vi "_CSMQFGV.vi"(6 "Operation":T3, 8 "Error in":errorcluster caption="Error in (no error)", 9 "create if not found? (T)":bool=TRUE, 11 "Name(\"\" to use uuid) in":string) -> (0 "Error out":errorcluster, 1 "Boolean":bool, 2 "Name":string[](array[string]), 3 "Array":T1[](array[typedef]))   [LabVIEW 2014, in "Communicable State Machine.lvlib"]
uses:
  Communicable State Machine.lvlib
  _CSMQFGVOPER.ctl
  _CSMObj.ctl
  Priority Queue/Priority Queue.lvclass
  Typedef/_CSM_MODE.ctl
  Typedef/_CSM Status Change Event Data.ctl
  Priority Queue/Priority Queue.lvclass/Priority Queue.ctl
  FGV-BroadcastRegistry/Operation-BroadcastRegistry.ctl
  FGV-BroadcastRegistry/global-CSMQ FGV Change Flag.vi
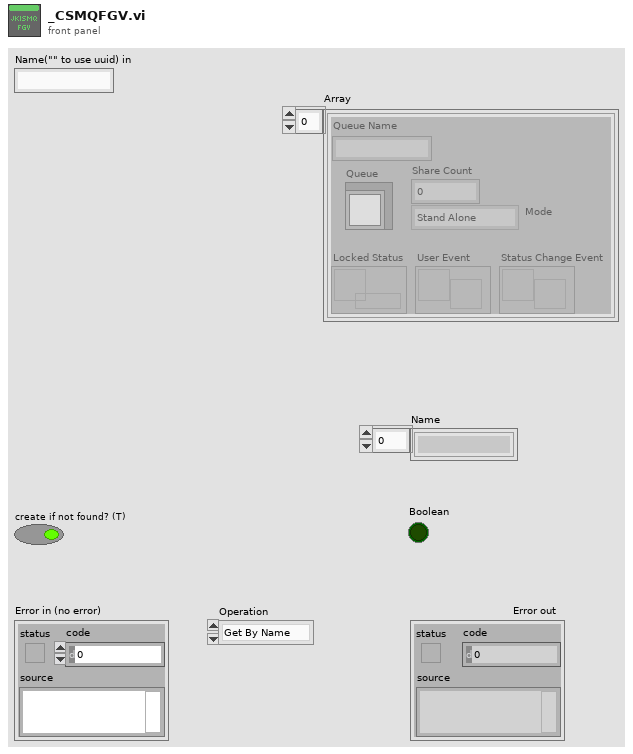
[diagram p1: front panel]
types:
  T1 = typedef "Communicable State Machine.lvlib/_CSMObj.ctl" = cluster{"Queue Name":string, "Mode":T2, "Share Count":i32, "Queue":refnum<class "Priority Queue.lvclass">, "Locked Status":refnum<data-value>, "User Event":refnum<user-event>, "Status Change Event":refnum<user-event>}
  T2 = typedef "Communicable State Machine.lvlib/_CSM_MODE.ctl" = enum16{"Stand Alone", "CSM", "Action Worker"}
  T3 = typedef "Communicable State Machine.lvlib/_CSMQFGVOPER.ctl" = enum16{"Get By Name", "List", "Check If Name Exists", "Release", "Module Status", "Create Status Event Handler", "Destroy Status Event Handler"}
  T4 = typedef "Communicable State Machine.lvlib/Operation-BroadcastRegistry.ctl" = enum16{"Delete Source Module", "Delete Target Module", "Remove Module", "Register", "Unregister", "Check"}
  T5 = typedef "Communicable State Machine.lvlib/_CSM Status Change Event Data.ctl" = cluster{"ModuleName":string, "Status":string, "Arguments":string}
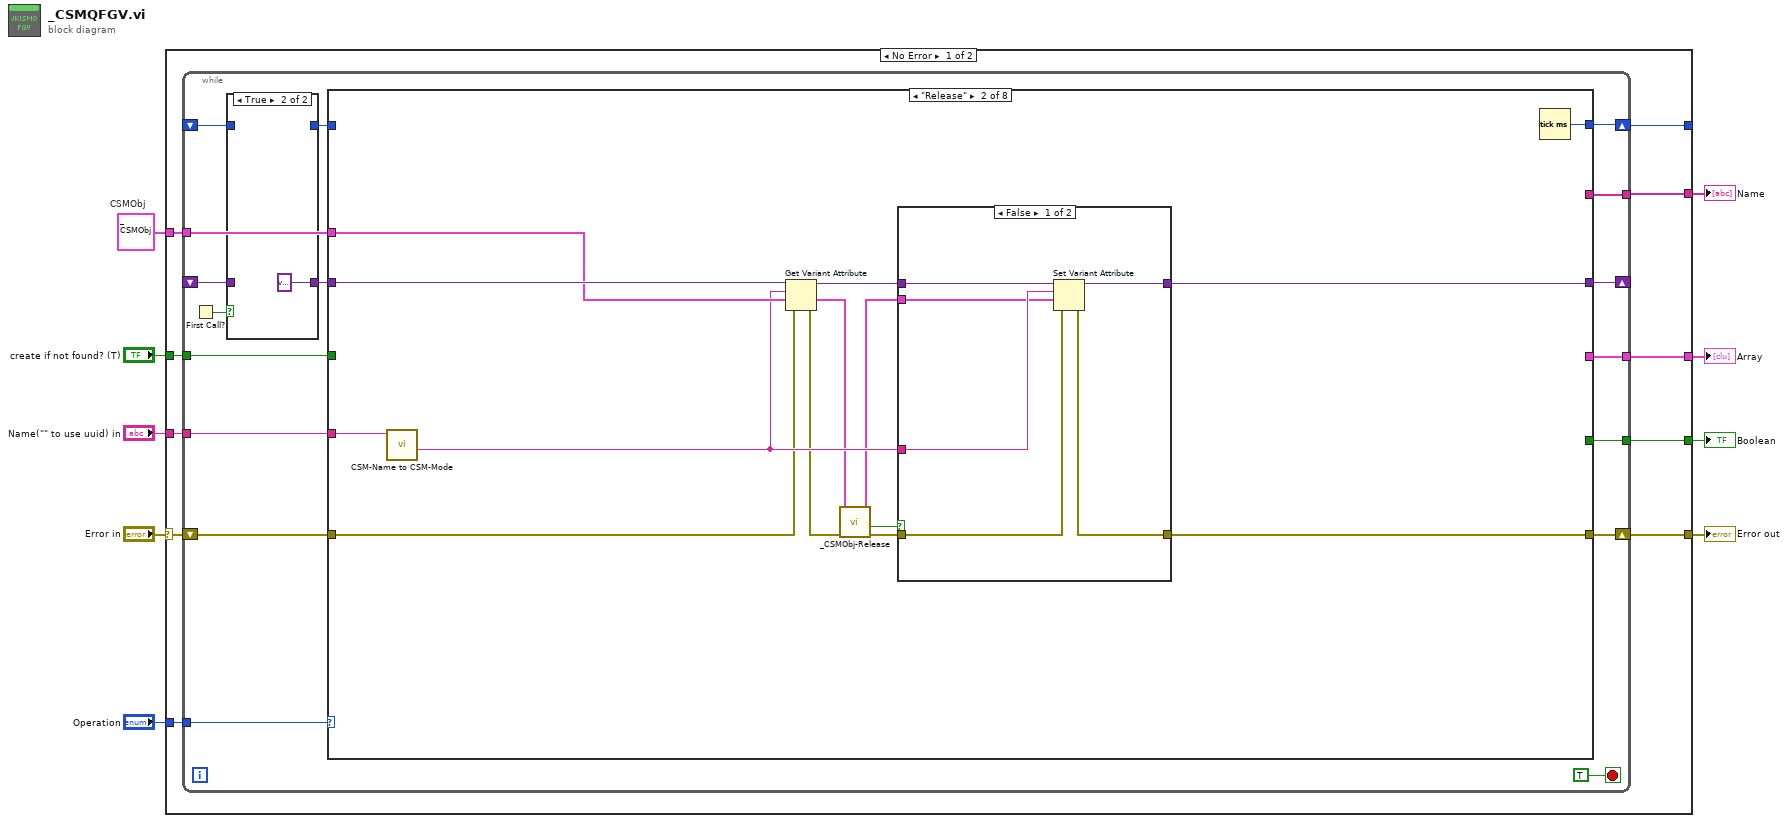
[diagram p0: block diagram]
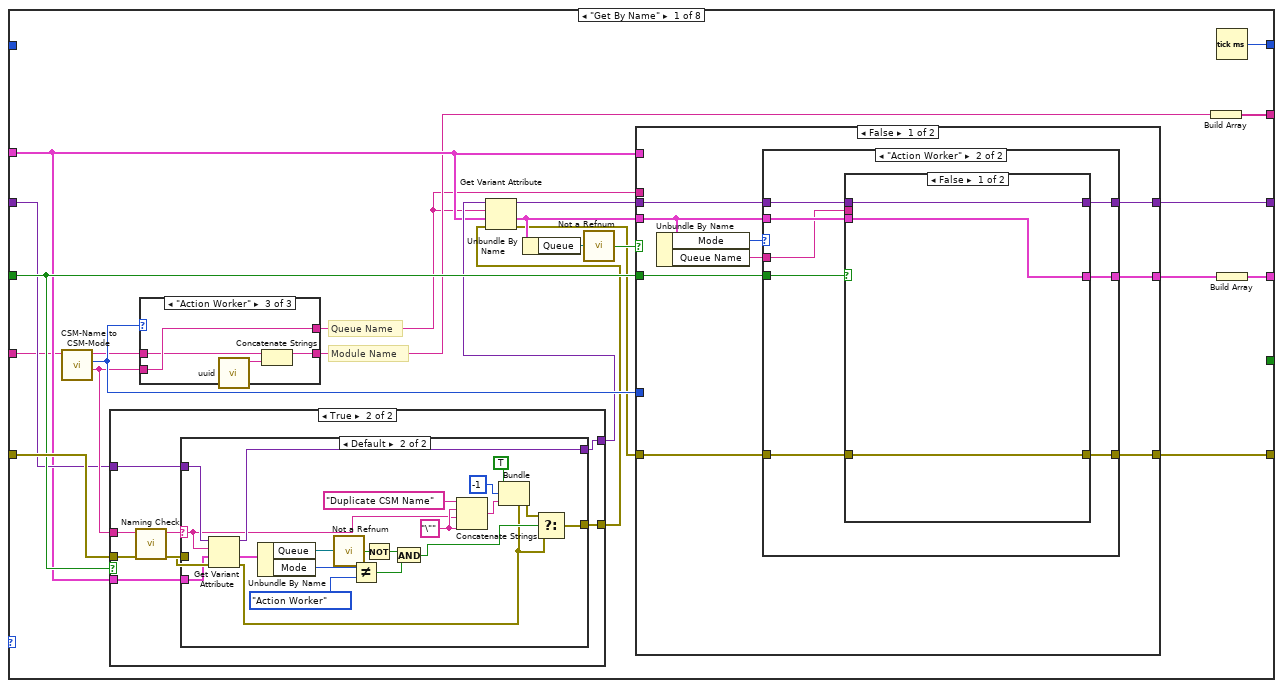
[diagram p3: hidden frame]
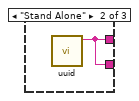
[diagram p7: hidden frame]
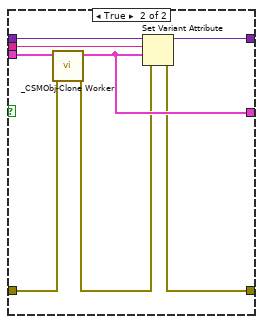
[diagram p9: hidden frame]
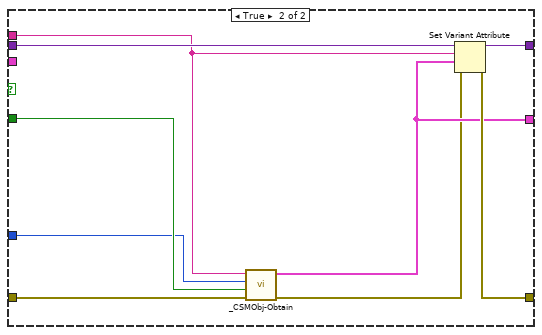
[diagram p10: hidden frame]
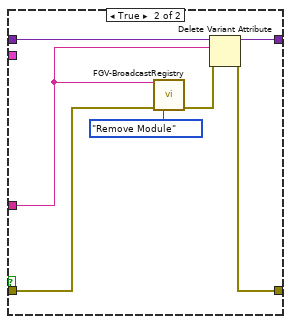
[diagram p11: hidden frame]
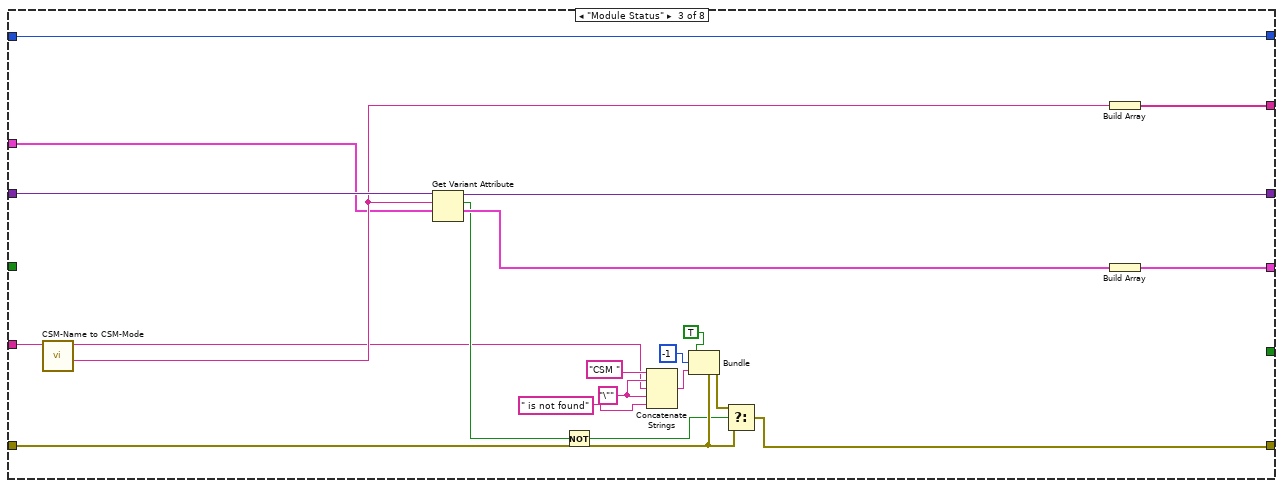
[diagram p12: hidden frame]
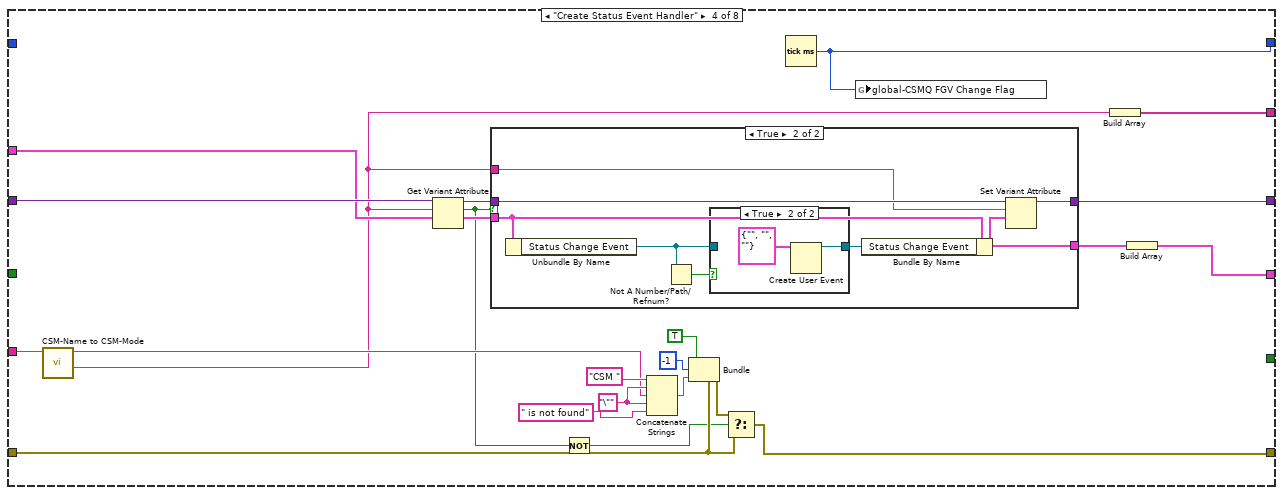
[diagram p13: hidden frame]
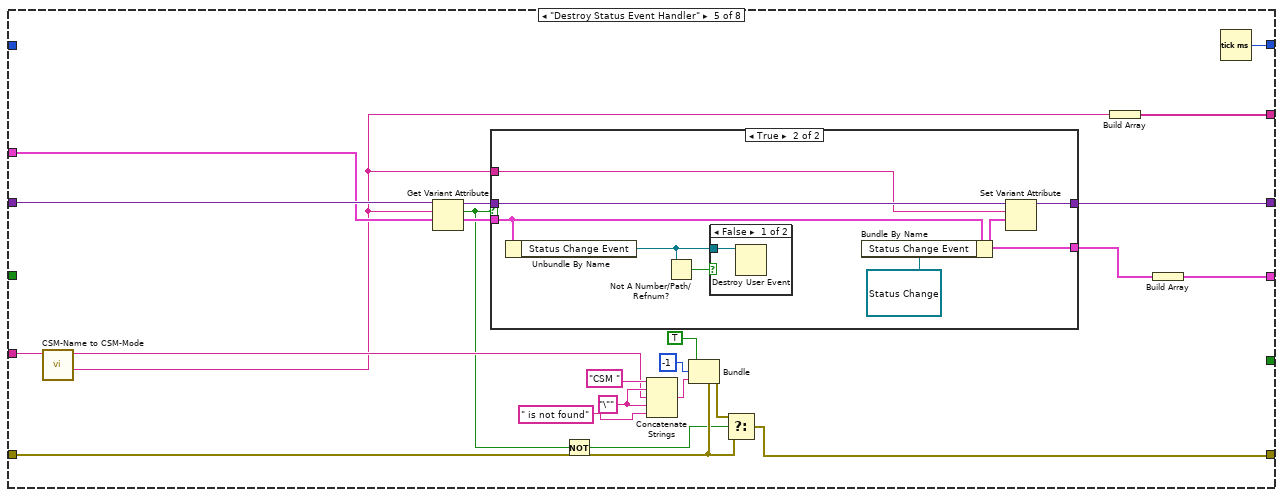
[diagram p16: hidden frame]
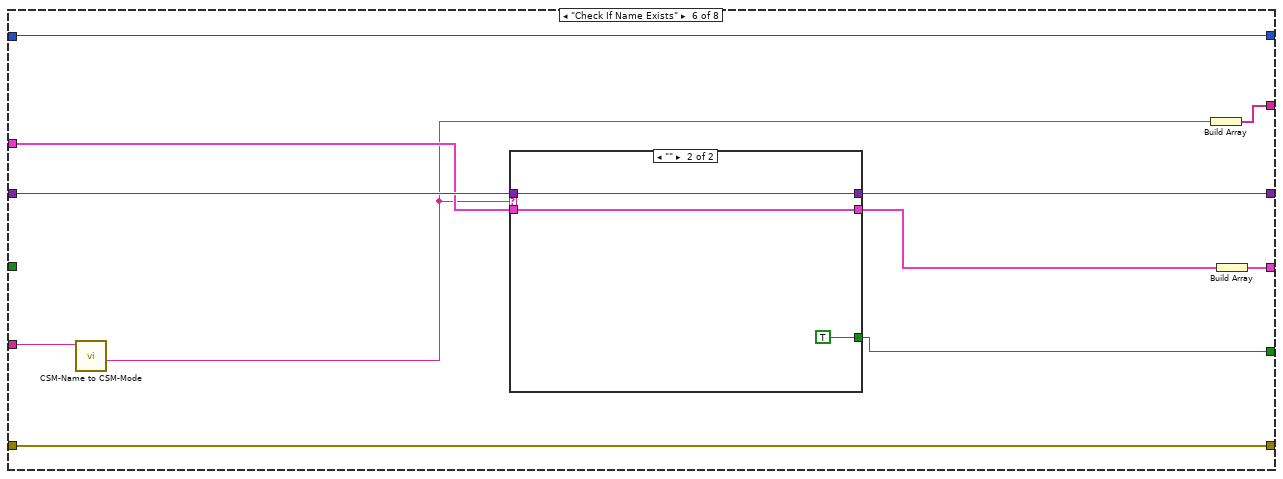
[diagram p19: hidden frame]
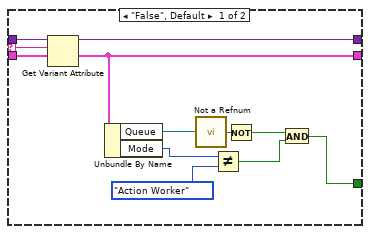
[diagram p20: hidden frame]
diagram:
  w3 = T1 {"Queue Name"="", "Mode"=enum."Stand Alone", "Share Count"=0, "Queue"=refnum, "Locked Status"=refnum, "User Event"=refnum, "Status Change Event"=refnum}  # CSMObj
  n1 = case shown="No Error" "Error in" {
    selector: "Error in" -> [w16 w340]
    tunnel: "Operation" -> [w19 _]
    tunnel: "Name(\"\" to use uuid) in" -> [w18 _]
    tunnel: "create if not found? (T)" -> [w17 _]
    tunnel: [w15 w340] -> w5
    tunnel: [w14 _] -> w4
    tunnel: w3 -> [w13 _]
    tunnel: [w12 _] -> w2
    tunnel: [w11 _] -> w1
    tunnel: [w10 _] -> _
    frame No Error {
      n2 = while {
        tunnel: w19 -> [w35]
        tunnel: w18 -> [w34]
        tunnel: w17 -> [w33]
        tunnel: [w32] -> w12
        shift-right: [w28] -> _
        shift-left: _ -> [w30]
        shift-right: [w26] -> w15
        shift-left: w16 -> [w27]
        tunnel: [w25] -> w14
        tunnel: w13 -> [w24]
        tunnel: [w23] -> w11
        shift-right: [w22] -> w10
        shift-left: _ -> [w20]
        stop <- TRUE stop-if-true
        n3 = First Call?() -> (First Call?: T/F=w31:bool)
        n4 = case shown="True" w31 {
          tunnel: [w38 variant] -> w29
          tunnel: w30 -> [w38 _]
          tunnel: [w37 _] -> w21
          tunnel: w20 -> [w37 _]
          frame False {
          }
          frame True {
          }
        }
        n5 = case shown="\"Release\"" w35 {
          tunnel: w34 -> [w42 w152 w188 w211 w247 w262 _ _]
          tunnel: w33 -> [w48 _ _ _ _ _ w293 _]
          tunnel: [w55 _ w185 w191 w227 w265 w288 _] -> w32
          tunnel: w29 -> [w47 w155 w189 w212 w248 w270 w301 w339]
          tunnel: [w60 w154 w187 w194 w230 w269 w300 w339] -> w28
          tunnel: w27 -> [w50 w149 w176 w203 w239 w267 w298 w338]
          tunnel: [w56 w148 w173 w201 w237 w267 w297 w338] -> w26
          tunnel: [w54 _ w183 w209 w245 w264 w289 _] -> w25
          tunnel: w24 -> [w45 w153 w181 w208 w244 w266 w299 _]
          tunnel: [_ _ _ _ _ w263 _ _] -> w23
          tunnel: w21 -> [_ _ w182 _ _ w260 w295 w337]
          tunnel: [w51 w150 w182 w190 w226 w260 w295 w337] -> w22
          frame "Get By Name" {
            # "Module Name"
            # "Queue Name"
            n6 = call "CSM-Name to CSM-Mode.vi"("String"=w42) -> ("Queue Name"=w49:string, "CSM Mode"=w53:T2, "String(dup)"=w52:string)  [unwired: 8 in]
            n7 = case shown="True" w48 {
              tunnel: w49 -> [_ w66]
              tunnel: [w64 w72] -> w44
              tunnel: w50 -> [w64 w68]
              tunnel: w47 -> [w63 w71]
              tunnel: [w63 w70] -> w46
              tunnel: w45 -> [_ w69]
              frame False {
              }
              frame True {
                n8 = call "Naming Check.vi"("error in (no error)"=w68, "Name(\"\" to use uuid)"=w66) -> ("error out"=w67:errorcluster, "Name(dup)"=w65:string)  [unwired: 8 in]
                n9 = case shown="Default" w65 {
                  selector: w65 -> [_ w75]
                  tunnel: [w73 w95] -> w72
                  tunnel: w67 -> [w73 w78]
                  tunnel: w71 -> [w74 w80]
                  tunnel: [w74 w79] -> w70
                  tunnel: w69 -> [_ w76]
                  frame "", "PostMessageAPI", "SendMessageAPI" {
                  }
                  frame Default {
                    w89 = "\"" ("string")
                    n10 = Get Variant Attribute(Variant=w80, name=w75, default value (empty Variant)=w76, error in=w78) -> (duplicate Variant=w79:variant, value=w82:T1, error out=w77:errorcluster)  [unwired: 1 out]
                    n11 = Unbundle By Name(w82) -> ("Queue"=w83:refnum<class "Priority Queue.lvclass">, "Mode"=w86:T2)
                    n12 = call "Not a Refnum.vi"("Priority Queue.lvclass"=w83) -> ("NaN/Path/Refnum?"=w84:bool)  [unwired: 4 in]
                    n13 = Not Equal?(x=w86, y=_CSM_MODE."Action Worker") -> (x != y?=w88:bool)
                    n14 = Not(x=w84) -> (.not. x?=w85:bool)
                    n15 = And(x=w85, y=w88) -> (x .and. y?=w81:bool)
                    n16 = Concatenate Strings("Duplicate CSM Name" ("String to Prepend to source (\"\")"), w89, w75, w89) -> (w90:string)
                    n17 = Bundle(cluster=w77, "status"=TRUE, "code"=-1, "source"=w90) -> (w94:errorcluster)
                    n18 = Select(t=w94, s=w81, f=w77) -> (s? t:f=w95:errorcluster)
                  }
                }
              }
            }
            n19 = case shown="\"Action Worker\"" w53 {
              tunnel: [w96 w97 w101] -> w40
              tunnel: [w96 w97 w98] -> w41
              tunnel: w52 -> [w96 _ w100]
              tunnel: w49 -> [_ _ w101]
              frame "CSM" {
              }
              frame "Stand Alone" {
                n20 = call "uuid.vi"() -> ("UUID"=w97:string)  [unwired: 11 in]
              }
              frame "Action Worker" {
                n21 = call "uuid.vi"() -> ("UUID"=w99:string)  [unwired: 11 in]
                n22 = Concatenate Strings(w100, w99) -> (w98:string)
              }
            }
            n23 = Get Variant Attribute(Variant=w46, name=w40, default value (empty Variant)=w45, error in=w44) -> (duplicate Variant=w61:variant, value=w59:T1, error out=w43:errorcluster)  [unwired: 1 out]
            n24 = Unbundle By Name(w59) -> ("Queue"=w58:refnum<class "Priority Queue.lvclass">)
            n25 = call "Not a Refnum.vi"("Priority Queue.lvclass"=w58) -> ("NaN/Path/Refnum?"=w57:bool)  [unwired: 4 in]
            n26 = case shown="False" w57 {
              tunnel: w48 -> [w102 w137]
              tunnel: [w108 w138] -> w62
              tunnel: w45 -> [_ _]
              tunnel: w61 -> [w109 w141]
              tunnel: [w110 w140] -> w60
              tunnel: w59 -> [w107 _]
              tunnel: w43 -> [w105 w135]
              tunnel: [w104 w139] -> w56
              tunnel: w53 -> [_ w133]
              tunnel: w40 -> [_ w134]
              frame False {
                n27 = Unbundle By Name(w107) -> ("Mode"=w106:T2, "Queue Name"=w103:string)
                n28 = case shown="\"Action Worker\"" w106 {
                  tunnel: [w113 w120] -> w110
                  tunnel: w109 -> [w113 w121]
                  tunnel: [w112 w118] -> w108
                  tunnel: w107 -> [w112 w119]
                  tunnel: w105 -> [w111 w117]
                  tunnel: [w111 w116] -> w104
                  tunnel: w103 -> [_ w115]
                  tunnel: w102 -> [_ w114]
                  frame Default {
                  }
                  frame "Action Worker" {
                    n29 = case shown="False" w114 {
                      tunnel: w121 -> [w124 w132]
                      tunnel: [w124 w131] -> w120
                      tunnel: w119 -> [w123 w130]
                      tunnel: [w123 w129] -> w118
                      tunnel: w117 -> [w122 w127]
                      tunnel: [w122 w126] -> w116
                      tunnel: w115 -> [_ w125]
                      frame False {
                      }
                      frame True {
                        n30 = call "_CSMObj-Clone Worker.vi"("Error in"=w127, "CSMObj in"=w130) -> ("Error out"=w128:errorcluster, "CSMObj out"=w129:T1)  [unwired: 8 in]
                        n31 = Set Variant Attribute(Variant=w132, name=w125, value=w129, error in=w128) -> (Variant out=w131:variant, error out=w126:errorcluster)  [unwired: 1 out]
                      }
                    }
                  }
                }
              }
              frame True {
                n32 = call "_CSMObj-Obtain.vi"("Error in"=w135, "create if not found? (T)"=w137, "Mode"=w133, "Queue Name"=w134) -> ("Error out"=w136:errorcluster, "CSMQ out"=w138:T1)  [unwired: 6 in]
                n33 = Set Variant Attribute(Variant=w141, name=w134, value=w138, error in=w136) -> (Variant out=w140:variant, error out=w139:errorcluster)  [unwired: 1 out]
              }
            }
            n34 = Build Array(w41) -> (w54:string[])
            n35 = Tick Count (ms)() -> (millisecond timer value=w51:u32)
            n36 = Build Array(w62) -> (w55:T1[])
          }
          frame "Release" {
            n37 = call "CSM-Name to CSM-Mode.vi"("String"=w152) -> ("Queue Name"=w151:string)  [unwired: 8 in, 2 out]
            n38 = Get Variant Attribute(Variant=w155, name=w151, default value (empty Variant)=w153, error in=w149) -> (duplicate Variant=w147:variant, value=w146:T1, error out=w142:errorcluster)  [unwired: 1 out]
            n39 = call "_CSMObj-Release.vi"("Error in"=w142, "CSMQ in"=w146) -> ("Error out"=w143:errorcluster, "Release?"=w145:bool, "CSMQ out"=w144:T1)  [unwired: 7 in]
            n40 = case shown="False" w145 {
              tunnel: w151 -> [w159 w165]
              tunnel: w147 -> [w161 w167]
              tunnel: [w160 w166] -> w154
              tunnel: w144 -> [w158 _]
              tunnel: w143 -> [w157 w164]
              tunnel: [w156 w162] -> w148
              frame False {
                n41 = Set Variant Attribute(Variant=w161, name=w159, value=w158, error in=w157) -> (Variant out=w160:variant, error out=w156:errorcluster)  [unwired: 1 out]
              }
              frame True {
                n42 = call "FGV-BroadcastRegistry.vi"("Source"=w165, "Error in"=w164, "Operation"=Operation-BroadcastRegistry."Remove Module") -> ("Error out"=w163:errorcluster)  [unwired: 10 in, 2 out]
                n43 = Delete Variant Attribute(4:w163, 6:w165, 7:w167) -> (0:w162:errorcluster, 3:w166:variant)  [unwired: 1 out]
              }
            }
            n44 = Tick Count (ms)() -> (millisecond timer value=w150:u32)
          }
          frame "Module Status" {
            w177 = "\"" ("string")
            n45 = call "CSM-Name to CSM-Mode.vi"("String"=w188) -> ("Queue Name"=w184:string, "String(dup)"=w171:string)  [unwired: 8 in, 1 out]
            n46 = Get Variant Attribute(Variant=w189, name=w184, default value (empty Variant)=w181) -> (duplicate Variant=w187:variant, found=w175:bool, value=w186:T1)  [unwired: 1 in, 1 out]
            n47 = Not(x=w175) -> (.not. x?=w174:bool)
            n48 = Concatenate Strings("CSM " ("String to Prepend to source (\"\")"), w177, w171, w177, " is not found" ("string")) -> (w178:string)
            n49 = Bundle(cluster=w176, "status"=TRUE, "code"=-1, "source"=w178) -> (w180:errorcluster)
            n50 = Select(t=w180, s=w174, f=w176) -> (s? t:f=w173:errorcluster)
            n51 = Build Array(w184) -> (w183:string[])
            n52 = Build Array(w186) -> (w185:T1[])
          }
          frame "Create Status Event Handler" {
            w204 = "\"" ("string")
            n53 = call "CSM-Name to CSM-Mode.vi"("String"=w211) -> ("Queue Name"=w193:string, "String(dup)"=w199:string)  [unwired: 8 in, 1 out]
            n54 = Get Variant Attribute(Variant=w212, name=w193, default value (empty Variant)=w208) -> (duplicate Variant=w195:variant, found=w196:bool, value=w210:T1)  [unwired: 1 in, 1 out]
            n55 = case shown="True" w196 {
              tunnel: w210 -> [w213 w217]
              tunnel: w195 -> [w214 w222]
              tunnel: [w214 w221] -> w194
              tunnel: w193 -> [_ w220]
              tunnel: [w213 w215] -> w192
              frame False {
              }
              frame True {
                n56 = Unbundle By Name(w217) -> ("Status Change Event"=w218:refnum<user-event>)
                n57 = Not A Number/Path/Refnum?(number/path/refnum=w218) -> (NaN/Path/Refnum?=w219:bool)
                n58 = case shown="True" w219 {
                  tunnel: w218 -> [w223 _]
                  tunnel: [w223 w224] -> w216
                  frame False {
                  }
                  frame True {
                    n59 = Create User Event(user event datatype=T5 {"ModuleName"="", "Status"="", "Arguments"=""} ("Status Message")) -> (user event=w224:refnum<user-event>)  [unwired: 1 in, 1 out]
                  }
                }
                n60 = Bundle By Name(cluster=w217, "Status Change Event"=w216) -> (w215:T1)
                n61 = Set Variant Attribute(Variant=w222, name=w220, value=w215) -> (Variant out=w221:variant)  [unwired: 1 in, 2 out]
              }
            }
            n62 = Not(x=w196) -> (.not. x?=w202:bool)
            n63 = Concatenate Strings("CSM " ("String to Prepend to source (\"\")"), w204, w199, w204, " is not found" ("string")) -> (w205:string)
            n64 = Bundle(cluster=w203, "status"=TRUE, "code"=-1, "source"=w205) -> (w207:errorcluster)
            n65 = Select(t=w207, s=w202, f=w203) -> (s? t:f=w201:errorcluster)
            n66 = Tick Count (ms)() -> (millisecond timer value=w190:u32)
            n67 = global write "global-CSMQ FGV Change Flag.vi" "global-CSMQ FGV Change Flag"(w190) -> ()
            n68 = Build Array(w193) -> (w209:string[])
            n69 = Build Array(w192) -> (w191:T1[])
          }
          frame "Destroy Status Event Handler" {
            w240 = "\"" ("string")
            n70 = call "CSM-Name to CSM-Mode.vi"("String"=w247) -> ("Queue Name"=w229:string, "String(dup)"=w235:string)  [unwired: 8 in, 1 out]
            n71 = Get Variant Attribute(Variant=w248, name=w229, default value (empty Variant)=w244) -> (duplicate Variant=w231:variant, found=w232:bool, value=w246:T1)  [unwired: 1 in, 1 out]
            n72 = case shown="True" w232 {
              tunnel: w246 -> [w249 w253]
              tunnel: w231 -> [w250 w258]
              tunnel: [w250 w257] -> w230
              tunnel: w229 -> [_ w256]
              tunnel: [w249 w252] -> w228
              frame False {
              }
              frame True {
                n73 = Unbundle By Name(w253) -> ("Status Change Event"=w254:refnum<user-event>)
                n74 = Not A Number/Path/Refnum?(number/path/refnum=w254) -> (NaN/Path/Refnum?=w255:bool)
                n75 = case shown="False" w255 {
                  tunnel: w254 -> [w259 _]
                  frame False {
                    n76 = Destroy User Event(user event=w259) -> ()  [unwired: 1 in, 1 out]
                  }
                  frame True {
                  }
                }
                n77 = Bundle By Name(cluster=w253, "Status Change Event"=refnum<user-event> refnum) -> (w252:T1)
                n78 = Set Variant Attribute(Variant=w258, name=w256, value=w252) -> (Variant out=w257:variant)  [unwired: 1 in, 2 out]
              }
            }
            n79 = Not(x=w232) -> (.not. x?=w238:bool)
            n80 = Concatenate Strings("CSM " ("String to Prepend to source (\"\")"), w240, w235, w240, " is not found" ("string")) -> (w241:string)
            n81 = Bundle(cluster=w239, "status"=TRUE, "code"=-1, "source"=w241) -> (w243:errorcluster)
            n82 = Select(t=w243, s=w238, f=w239) -> (s? t:f=w237:errorcluster)
            n83 = Build Array(w229) -> (w245:string[])
            n84 = Build Array(w228) -> (w227:T1[])
            n85 = Tick Count (ms)() -> (millisecond timer value=w226:u32)
          }
          frame "Check If Name Exists" {
            n86 = call "CSM-Name to CSM-Mode.vi"("String"=w262) -> ("Queue Name"=w261:string)  [unwired: 8 in, 2 out]
            n87 = case shown="\"\"" w261 {
              selector: w261 -> [w279 _]
              tunnel: w270 -> [w282 w285]
              tunnel: [w281 w285] -> w269
              tunnel: [w278 w283] -> w268
              tunnel: w266 -> [w280 w283]
              tunnel: [w274 TRUE] -> w263
              frame "False", Default {
                n88 = Get Variant Attribute(Variant=w282, name=w279, default value (empty Variant)=w280) -> (duplicate Variant=w281:variant, value=w278:T1)  [unwired: 1 in, 2 out]
                n89 = Unbundle By Name(w278) -> ("Queue"=w277:refnum<class "Priority Queue.lvclass">, "Mode"=w273:T2)
                n90 = call "Not a Refnum.vi"("Priority Queue.lvclass"=w277) -> ("NaN/Path/Refnum?"=w276:bool)  [unwired: 4 in]
                n91 = Not Equal?(x=w273, y=_CSM_MODE."Action Worker") -> (x != y?=w271:bool)
                n92 = Not(x=w276) -> (.not. x?=w275:bool)
                n93 = And(x=w275, y=w271) -> (x .and. y?=w274:bool)
              }
              frame "" {
              }
            }
            n94 = Build Array(w261) -> (w264:string[])
            n95 = Build Array(w268) -> (w265:T1[])
          }
          frame "List" {
            n96 = feedback-in #1(w295) -> ()
            n97 = feedback #1() -> (w296:u32)  [unwired: 1 in]
            n98 = feedback #2() -> (w294:bool)  [unwired: 1 in]
            n99 = feedback-in #2(w293) -> ()
            n100 = Not Equal?(x=w295, y=w296) -> (x != y?=w291:bool)
            n101 = Not Equal?(x=w293, y=w294) -> (x != y?=w292:bool)
            n102 = Or(x=w291, y=w292) -> (x .or. y?=w290:bool)
            n103 = feedback #3() -> (w286:string[])  [unwired: 1 in]
            n104 = feedback #4() -> (w287:T1[])  [unwired: 1 in]
            n105 = case shown="True" w290 {
              tunnel: w301 -> [w303 w318]
              tunnel: [w303 w317] -> w300
              tunnel: w299 -> [_ w315]
              tunnel: [w304 w311] -> w289
              tunnel: [w305 w310] -> w288
              tunnel: w298 -> [w302 w308]
              tunnel: [w302 w307] -> w297
              tunnel: w293 -> [_ w306]
              tunnel: w287 -> [w305 _]
              tunnel: w286 -> [w304 _]
              frame False {
              }
              frame True {
                n106 = disable-structure shown="Enabled" {
                  disable-tunnel: w315 -> [w336 _]
                  disable-tunnel: [w335 _] -> w314
                  frame Disabled {
                    n107 = Build Array(w336) -> (w335:T1[])
                  }
                  frame Enabled {
                  }
                }
                n108 = Get Variant Attribute(Variant=w318, error in=w308) -> (duplicate Variant=w317:variant, names=w312:string[], values=w316:variant[], error out=w309:errorcluster)  [unwired: 2 in]
                n109 = Variant To Data(error in=w309, type=w314, Variant=w316) -> (data=w313:T1[], error out=w307:errorcluster)
                n110 = for {
                  tunnel: w313 -> [w331] mode=indexing
                  tunnel: w312 -> [w322] mode=indexing
                  tunnel: [w322] -> w311 mode=indexing if=w323
                  tunnel: [w331] -> w310 mode=indexing if=w323
                  tunnel: w306 -> [w324]
                  n111 = Unbundle By Name(w331) -> ("Queue"=w330:refnum<class "Priority Queue.lvclass">, "Mode"=w326:T2)
                  n112 = case shown="\"Stand Alone\"" w326 {
                    tunnel: [w332 TRUE] -> w325
                    tunnel: w324 -> [w333 _]
                    frame "Stand Alone" {
                      n113 = Not(x=w333) -> (.not. x?=w332:bool)
                    }
                    frame Default {
                    }
                  }
                  n114 = call "Not a Refnum.vi"("Priority Queue.lvclass"=w330) -> ("NaN/Path/Refnum?"=w329:bool)  [unwired: 4 in]
                  n115 = Not(x=w329) -> (.not. x?=w327:bool)
                  n116 = Match Pattern(string=w322, regular expression="^-") -> (offset past match=w320:i32)  [unwired: 1 in, 3 out]
                  n117 = And(x=w327, y=w325) -> (x .and. y?=w328:bool)
                  n118 = Less Than 0?(x=w320) -> (x < 0?=w319:bool)
                  n119 = And(x=w319, y=w328) -> (x .and. y?=w323:bool)
                }
              }
            }
            n120 = feedback-in #3(w289) -> ()
            n121 = feedback-in #4(w288) -> ()
          }
          frame Default {
          }
        }
      }
    }
    frame Error {
    }
  }
  "Error out" <- w5
  "Name" <- w4
  "Array" <- w2
  "Boolean" <- w1
